vi "create channels from assembly.vi"(8 "error in":errorcluster, 9 "assembly definition":T1, 10 "engine configuration in":refnum<class "engine configuration.lvclass">, 11 "EthernetIP configuration in":refnum<class "EthernetIP configuration.lvclass">) -> (0 "error out":errorcluster, 2 "engine configuration out":refnum<class "engine configuration.lvclass">, 3 "EthernetIP configuration out":refnum<class "EthernetIP configuration.lvclass">)   [LabVIEW 2013, in "EthernetIP editor node.lvclass"]
uses:
  EthernetIP editor node.lvclass
  <vilib>/NI/TBM Modules/Ethernet IP/configuration/assembly definition.ctl
  <vilib>/NI/TBM Modules/Ethernet IP/configuration/assembly type.ctl
  <vilib>/NI/Tag Bus/tag/Data Type.ctl
  <vilib>/NI/Module Execution Interface/Engine Configuration/engine configuration.lvclass
  <vilib>/NI/TBM Modules/Ethernet IP/configuration/EthernetIP configuration.lvclass
  <vilib>/NI/TBM Modules/Ethernet IP/configuration/EthernetIP configuration.lvclass/EthernetIP configuration.ctl
  <vilib>/NI/Tag Bus Module Framework/root configuration/TBM configuration.lvclass/TBM configuration.ctl
  <vilib>/NI/TBM Modules/Ethernet IP/channel/EthernetIP Channel.lvclass/EthernetIP Channel.ctl
  <vilib>/NI/TBM Modules/Ethernet IP/channel/Read Instance ID.vi
  <vilib>/NI/TBM Modules/Ethernet IP/channel/Read byte index.vi
  <vilib>/NI/Tag Bus Module Framework/root configuration/Read instance name.vi
  <vilib>/NI/TBM Modules/Ethernet IP/configuration/read eip channels.vi
  <vilib>/NI/TBM Modules/Ethernet IP/configuration/Read assemblies.vi
  <vilib>/NI/Tag Bus Module Framework/root configuration/create GUID.vi
  <vilib>/NI/TBM Modules/Ethernet IP/channel/EthernetIP Channel.lvclass
  <vilib>/NI/Tag Bus/tag/tag descriptor.lvclass
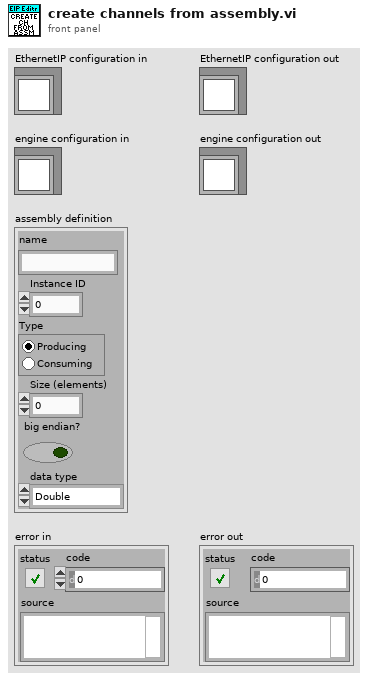
[diagram p1: front panel]
types:
  T1 = typedef "EthernetIP configuration.lvclass/assembly definition.ctl" = cluster{"name":string, "Instance ID":u32, "Type":T2, "Size (elements)":u32, "big endian?":bool, "data type":T3}
  T2 = typedef "EthernetIP configuration.lvclass/assembly type.ctl" = enum32{"Producing", "Consuming"}
  T3 = typedef "tag bus.lvlib/tag descriptor.lvclass/Data Type.ctl" = enum16{"Double", "Single", "I64", "I32", "I16", "I8", "U64", "U32", "U16", "U8", "Boolean", "String", "Array of Double", "Array of Single", "Array of I64", "Array of I32", "Array of I16", "Array of I8", "Array of U64", "Array of U32", "Array of U16", "Array of U8", "Array of Boolean", "Array of String"}
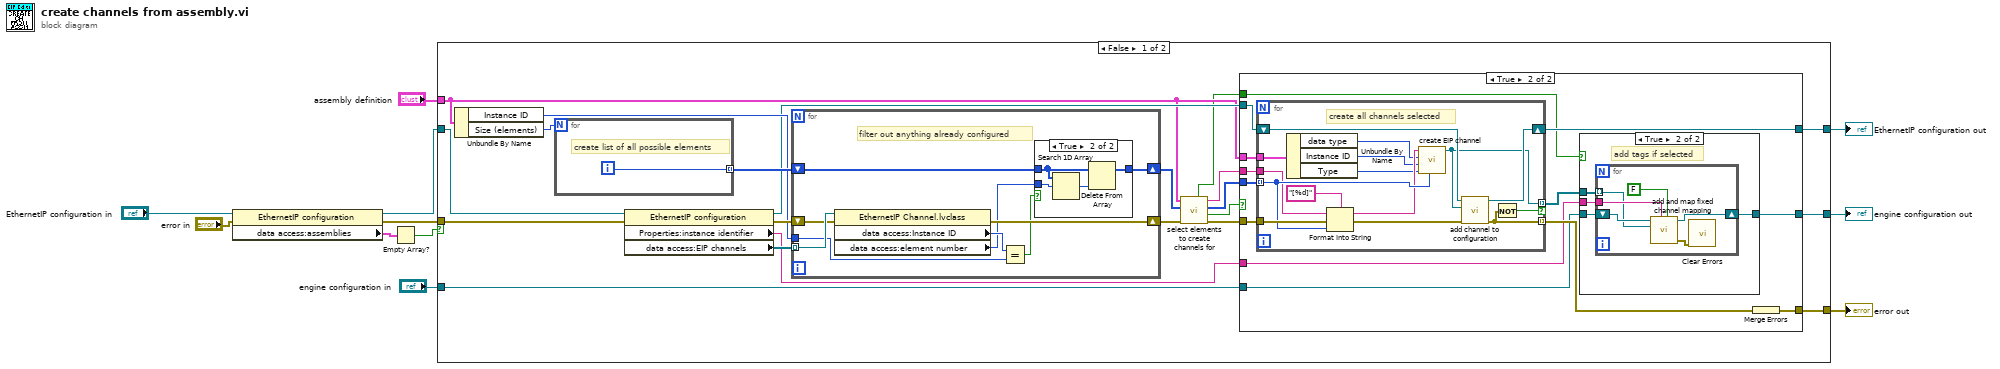
[diagram p0: block diagram]
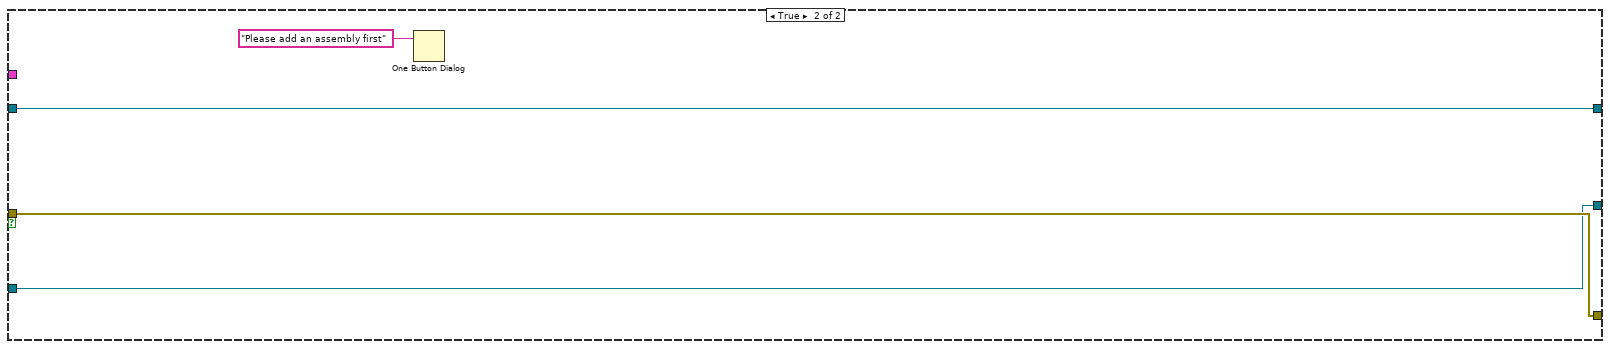
[diagram p5: hidden frame]
diagram:
  n1 = property class="EthernetIP configuration"(reference="EthernetIP configuration in", error in="error in") -> (reference out=w7:refnum<class "EthernetIP configuration.lvclass">, error out=w6:errorcluster, "data access:assemblies"=w9:T1[])
  n2 = Empty Array?(array=w9) -> (empty?=w8:bool)
  n3 = case shown="False" w8 {
    tunnel: w7 -> [w32 w93]
    tunnel: w6 -> [w31 w92]
    tunnel: [w22 w93] -> w5
    tunnel: [w19 w92] -> w4
    tunnel: "assembly definition" -> [w16 _]
    tunnel: [w14 w90] -> w1
    tunnel: "engine configuration in" -> [w13 w90]
    frame False {
      n4 = Unbundle By Name(w16) -> ("Instance ID"=w26:u32, "Size (elements)"=w30:u32)
      n5 = for {
        N: w30 -> [_]
        tunnel: [w89] -> w29 mode=indexing
        i -> [w89]
        # "create list of all possible elements"
      }
      n6 = property class="EthernetIP configuration"(reference=w32, error in=w31) -> (reference out=w21:refnum<class "EthernetIP configuration.lvclass">, error out=w27:errorcluster, "Properties:instance identifier"=w12:string, "data access:EIP channels"=w28:refnum<class "EthernetIP Channel.lvclass">[])
      n7 = for {
        shift-right: [w75] -> w24
        shift-left: w29 -> [w77]
        tunnel: w28 -> [w83] mode=indexing
        shift-right: [w81] -> w25
        shift-left: w27 -> [w82]
        tunnel: w26 -> [w79]
        # "filter out anything already configured"
        n8 = property class="EthernetIP Channel.lvclass"(reference=w83, error in=w82) -> (error out=w81:errorcluster, "data access:Instance ID"=w80:u32, "data access:element number"=w76:i32)  [unwired: 1 out]
        n9 = Equal?(x=w80, y=w79) -> (x = y?=w78:bool)
        n10 = case shown="True" w78 {
          tunnel: w77 -> [w84 w87]
          tunnel: w76 -> [_ w88]
          tunnel: [w84 w86] -> w75
          frame False {
          }
          frame True {
            n11 = Search 1D Array(1D array=w87, element=w88) -> (index of element=w85:i32)  [unwired: 1 in]
            n12 = Delete From Array(array=w87, index=w85) -> (array with subset deleted=w86:i32[])  [unwired: 1 in, 1 out]
          }
        }
      }
      n13 = call "select elements to create channels for.vi"("error in"=w25, "allowable channels"=w24, "assembly definition"=w16) -> ("error out"=w20:errorcluster, "cancelled?"=w23:bool, "channels to create"=w18:i32[], "base channame"=w17:string, "create tags"=w15:bool)  [unwired: 4 in]
      n14 = case shown="True" w23 {
        tunnel: [w35 w45] -> w22
        tunnel: w21 -> [w35 w46]
        tunnel: w20 -> [w34 w48]
        tunnel: [w34 w42] -> w19
        tunnel: w18 -> [_ w44]
        tunnel: w17 -> [_ w43]
        tunnel: w16 -> [_ w41]
        tunnel: w15 -> [_ w40]
        tunnel: [w33 w39] -> w14
        tunnel: w13 -> [w33 w38]
        tunnel: w12 -> [_ w37]
        frame False {
        }
        frame True {
          n15 = for {
            shift-right: [w74] -> w45
            shift-left: w46 -> [w73]
            tunnel: w44 -> [w71] mode=indexing
            tunnel: w43 -> [w68]
            tunnel: w48 -> [w72]
            tunnel: [w61] -> w47 mode=indexing
            tunnel: w41 -> [w66]
            tunnel: [w62] -> w36 mode=indexing if=w60
            # "create all channels selected"
            n16 = Unbundle By Name(w66) -> ("data type"=w65:T3, "Instance ID"=w64:u32, "Type"=w63:T2)
            n17 = Format Into String(format string="[%d]", initial string=w68, error in=w72, w71) -> (resulting string=w67:string, error out=w70:errorcluster)
            n18 = call <vilib>:"create EIP channel.vi"("element"=w71, "Type"=w63, "Instance ID"=w64, "data type"=w65, "name"=w67) -> ("EthernetIP Channel out"=w62:refnum<class "EthernetIP Channel.lvclass">)  [unwired: 6 in]
            n19 = call <vilib>:"add channel to configuration.vi"("error in"=w70, "TBM channel in"=w62, "EthernetIP configuration in"=w73) -> ("error out"=w61:errorcluster, "EthernetIP configuration out"=w74:refnum<class "EthernetIP configuration.lvclass">)  [unwired: 7 in]
            n20 = Not(x=w61) -> (.not. x?=w60:bool)
          }
          n21 = case shown="True" w40 {
            tunnel: [w49 w52] -> w39
            tunnel: w38 -> [w49 w53]
            tunnel: w37 -> [_ w51]
            tunnel: w36 -> [_ w50]
            frame False {
            }
            frame True {
              # "add tags if selected"
              n22 = for {
                shift-right: [w57] -> w52
                shift-left: w53 -> [w59]
                tunnel: w51 -> [w56]
                tunnel: w50 -> [w54] mode=indexing
                n23 = call <vilib>:"add and map fixed channel mapping.vi"("set module as owner"=FALSE, "module instance"=w56, "fixed channel"=w54, "engine configuration in"=w59) -> ("error out"=w58:errorcluster, "engine configuration out"=w57:refnum<class "engine configuration.lvclass">)  [unwired: 6 in]
                n24 = call <vilib>:"Clear Errors.vi"("error in (no error)"=w58) -> ()  [unwired: 6 in, 1 out]
              }
            }
          }
          n25 = Merge Errors(w47) -> (w42:errorcluster)
        }
      }
    }
    frame True {
      n26 = One Button Dialog(message="Please add an assembly first") -> ()  [unwired: 1 in, 1 out]
    }
  }
  "engine configuration out" <- w1
  "EthernetIP configuration out" <- w5
  "error out" <- w4
